vi "After Launch Init Core.vi"(8 "error in (no error)":errorcluster, 11 "CS++Scope in":refnum<class "CS++Scope.lvclass">) -> (0 "error out":errorcluster, 3 "CS++Scope out":refnum<class "CS++Scope.lvclass">)   [LabVIEW 2015, in "CS++Scope.lvlib" / "CS++Scope.lvclass"]
doc: "Use <b>Pre Launch init.vi</b> method for sanity checks that are supposed to prevent the actor from launching if they fail. Use <B>this</B> method instead to initialize this actor when it has been activated. A corresponding high priority message will become dispatched before the <B>Actor Core.vi</b> is called.\n\n<b>Derived classed should call the parent methode first</b> and their own initialization code after.\n\nRefer also to the ongoing discussion at https://decibel.ni.com/content/message/57394#57394."
uses:
  CS++Scope.lvclass
  CSPP_Core/Classes/CS++ProcessVariables/ProcessVariable/PV.lvclass
  <vilib>/ActorFramework/Actor/Actor.lvclass
  CSPP_Core/Classes/CS++ProcessVariables/PVConnection/PVConnection.lvclass
  CSPP_Core/Actors/CS++DeviceActor/CS++DeviceActor.lvclass
  <vilib>/ActorFramework/Batch Msg/Batch Msg.lvclass
  CS++Scope Messages/Configure Acquisition Type Msg/Configure Acquisition Type Msg.lvclass
  CS++Scope Messages/Configure Acquisition Record Msg/Configure Acquisition Record Msg.lvclass
  CS++Scope Messages/Configure Channel Msg/Configure Channel Msg.lvclass
  CS++Scope Messages/Configure Trigger Msg/Configure Trigger Msg.lvclass
  CS++Scope Messages/Configure Trigger Modifier [TM] Msg/Configure Trigger Modifier [TM] Msg.lvclass
  CS++Scope Messages/Configure Edge Trigger Source Msg/Configure Edge Trigger Source Msg.lvclass
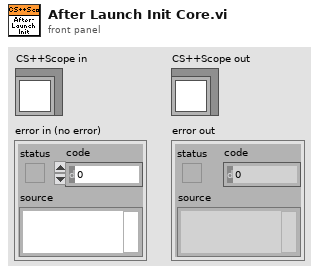
[diagram p1: front panel]
types:
  T1 = cluster{"Read Access":enum8{"Allowed", "Required", "None"}, "Write Access":enum8{"Allowed", "Required", "None"}}
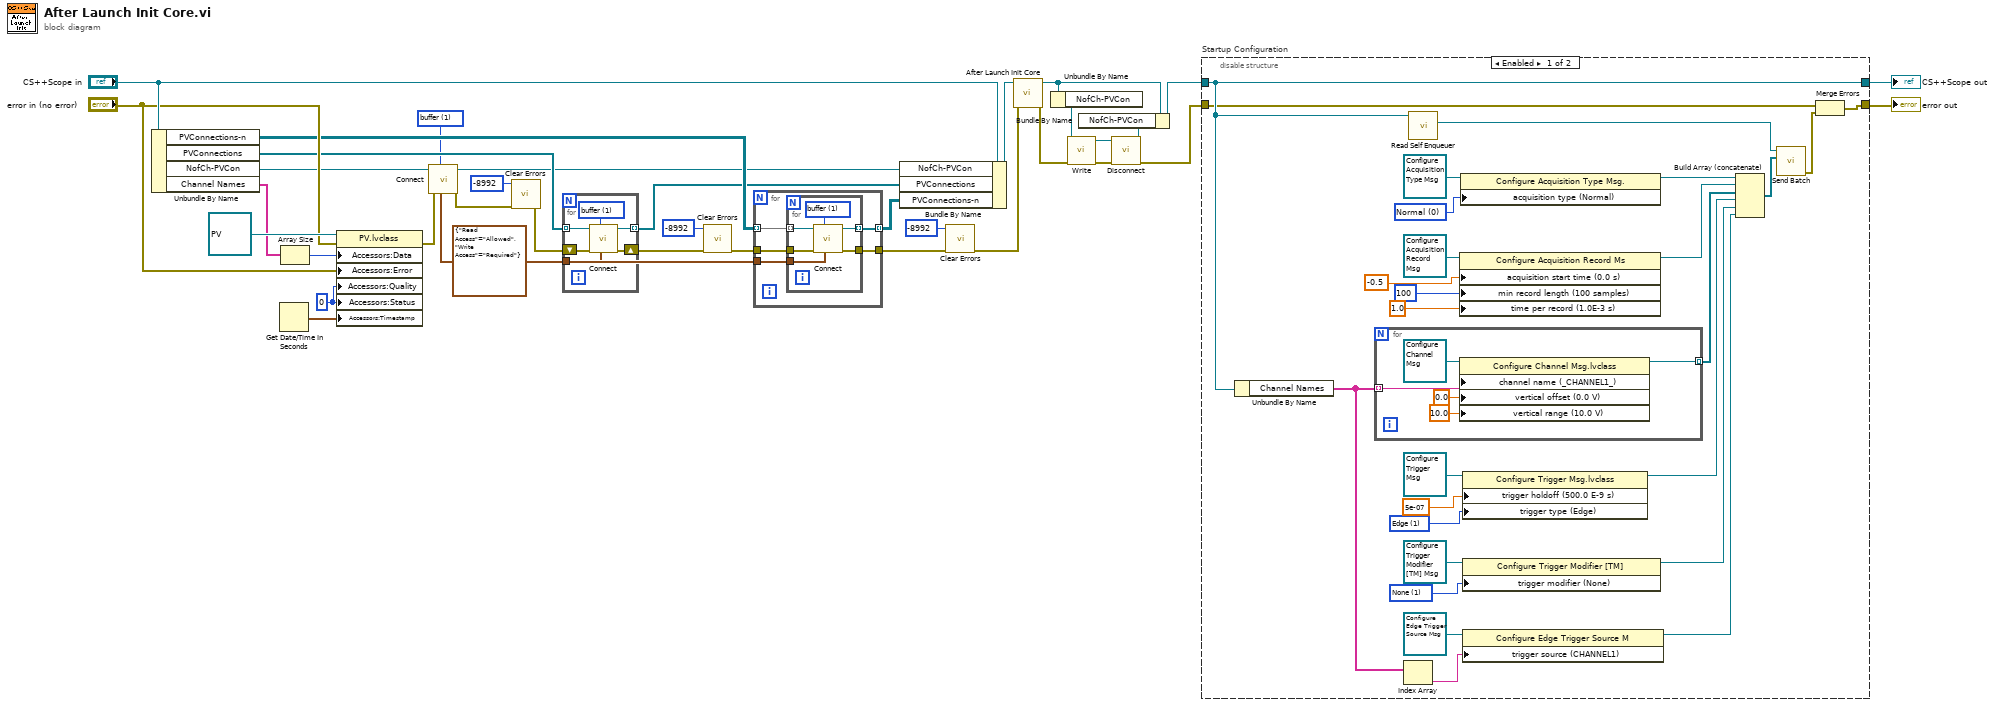
[diagram p0: block diagram]
diagram:
  w15 = u16 1 items=["commit", "buffer"] ("Mode (commit)")
  w20 = T1 {"Read Access"=enum."Allowed", "Write Access"=enum."Required"} ("Access (R/W allowed)")
  w26 = 0 ("Status")
  n1 = Unbundle By Name("CS++Scope in") -> ("PVConnections-n"=w29:refnum<class "PVConnection.lvclass">[][], "PVConnections"=w30:refnum<class "PVConnection.lvclass">[], "NofCh-PVCon"=w32:refnum<class "PVConnection.lvclass">, "Channel Names"=w23:string[])
  n2 = Get Date/Time In Seconds() -> (seconds since 1Jan1904=w25:timestamp)
  n3 = Array Size(array=w23) -> (size(s)=w24:i32)
  n4 = property class="PV.lvclass"(reference=refnum<class "PV.lvclass"> refnum ("CS++ProcessVariables.lvlib:PV.lvclass"), error in="error in (no error)", "Accessors:Data"=w24, "Accessors:Error"="error in (no error)", "Accessors:Quality"=w26, "Accessors:Status"=w26, "Accessors:Timestamp"=w25) -> (error out=w31:errorcluster)  [unwired: 1 out]
  n5 = call "Connect.vi"("Access (R/W allowed)"=w20, "Mode (buffer)"=w15, "Error In"=w31, "PVConnection in"=w32) -> ("Error Out"=w13:errorcluster, "PVConnection out"=w16:refnum<class "PVConnection.lvclass">)  [unwired: 6 in]
  n6 = call <vilib>:"Clear Errors.vi"("error in (no error)"=w13, "specific error code to clear (0: all)"=-8992) -> ("error out"=w12:errorcluster)  [unwired: 4 in, 1 out]
  n7 = for {
    tunnel: w30 -> [w42] mode=indexing
    shift-right: [w40] -> w10
    shift-left: w12 -> [w41]
    tunnel: [w39] -> w27 mode=indexing
    tunnel: w20 -> [w38]
    w37 = u16 1 items=["commit", "buffer"] ("Mode (commit)")
    n8 = call "Connect.vi"("Access (R/W allowed)"=w38, "Mode (buffer)"=w37, "Error In"=w41, "PVConnection in"=w42) -> ("Error Out"=w40:errorcluster, "PVConnection out"=w39:refnum<class "PVConnection.lvclass">)  [unwired: 6 in]
  }
  n9 = call <vilib>:"Clear Errors.vi"("error in (no error)"=w10, "specific error code to clear (0: all)"=-8992) -> ("error out"=w9:errorcluster)  [unwired: 4 in, 1 out]
  n10 = for {
    tunnel: w29 -> [w47] mode=indexing
    tunnel: [w44] -> w28 mode=indexing
    tunnel: w20 -> [w43]
    tunnel: w9 -> [w46]
    tunnel: [w45] -> w18
    n11 = for {
      tunnel: w47 -> [w53] mode=indexing
      tunnel: [w50] -> w44 mode=indexing
      tunnel: w43 -> [w49]
      tunnel: w46 -> [w52]
      tunnel: [w51] -> w45
      w48 = u16 1 items=["commit", "buffer"] ("Mode (commit)")
      n12 = call "Connect.vi"("Access (R/W allowed)"=w49, "Mode (buffer)"=w48, "Error In"=w52, "PVConnection in"=w53) -> ("Error Out"=w51:errorcluster, "PVConnection out"=w50:refnum<class "PVConnection.lvclass">)  [unwired: 6 in]
    }
  }
  n13 = Bundle By Name(cluster="CS++Scope in", "NofCh-PVCon"=w16, "PVConnections"=w27, "PVConnections-n"=w28) -> (w35:refnum<class "CS++Scope.lvclass">)
  n14 = call <vilib>:"Clear Errors.vi"("error in (no error)"=w18, "specific error code to clear (0: all)"=-8992) -> ("error out"=w17:errorcluster)  [unwired: 4 in, 1 out]
  n15 = call-parent "After Launch Init Core.vi"("error in (no error)"=w17, "CS++DeviceActor in"=w35) -> ("error out"=w5:errorcluster, "CS++DeviceActor out"=w3:refnum<class "CS++Scope.lvclass">)  [unwired: 8 in]
  n16 = Unbundle By Name(w3) -> ("NofCh-PVCon"=w6:refnum<class "PVConnection.lvclass">)
  n17 = call "Write.vi"("error in (no error)"=w5, "PVConnection in"=w6) -> ("error out"=w7:errorcluster, "PVConnection out"=w8:refnum<class "PVConnection.lvclass">)  [unwired: 8 in]
  n18 = call "Disconnect.vi"("error in (no error)"=w7, "PVConnection in"=w8) -> ("error out"=w4:errorcluster, "PVConnection out"=w1:refnum<class "PVConnection.lvclass">)  [unwired: 8 in]
  n19 = Bundle By Name(cluster=w3, "NofCh-PVCon"=w1) -> (w2:refnum<class "CS++Scope.lvclass">)
  n20 = disable-structure "Startup Configuration" shown="Enabled" {
    disable-tunnel: w4 -> [w54 w85]
    disable-tunnel: [w56 w85] -> w21
    disable-tunnel: [w57 w86] -> w22
    disable-tunnel: w2 -> [w57 w86]
    frame Enabled {
      w68 = 1 items=["None"=1, "Auto"=2, "Auto Level"=3] ("trigger modifier (None)")
      w66 = 1 items=["Edge"=1, "TV"=5, "Runt"=3, "Glitch"=4, "Width"=2, "AC Line"=7, "Immediate"=6] ("trigger type (Edge)")
      w59 = 0 items=["Normal", "Peak Detect", "High Resolution", "Envelope", "Average"] ("acquisition type (Normal)")
      n21 = Unbundle By Name(w57) -> ("Channel Names"=w79:string[])
      n22 = for {
        tunnel: [w83] -> w73 mode=indexing
        tunnel: w79 -> [w82] mode=indexing
        n23 = property class="Configure Channel Msg.lvclass"(reference=refnum<class "Configure Channel Msg.lvclass"> refnum ("CS++Scope.lvlib:Configure Channel Msg.lvclass"), "channel name (_CHANNEL1_)"=w82, "vertical offset (0.0 V)"=dbl[unit] 0.0, "vertical range (10.0 V)"=dbl[unit] 10.0) -> (reference out=w83:refnum<class "Configure Channel Msg.lvclass">)  [unwired: 1 in, 1 out]
      }
      n24 = Index Array(array=w79) -> (element=w70:string)  [unwired: 1 in]
      n25 = call <vilib>:"Read Self Enqueuer.vi"("Actor"=w57) -> ("Self Enqueuer"=w78:refnum<class "Message Enqueuer.lvclass">)  [unwired: 10 in]
      n26 = property class="Configure Acquisition Record Ms"(reference=refnum<class "Configure Acquisition Record Msg.lvclass"> refnum ("CS++Scope.lvlib:Configure Acquisition Record Msg.lvclass"), "acquisition start time (0.0 s)"=dbl[unit] -0.5, "min record length (100 samples)"=100, "time per record (1.0E-3 s)"=dbl[unit] 1.0) -> (reference out=w72:refnum<class "Configure Acquisition Record Msg.lvclass">)  [unwired: 1 in, 1 out]
      n27 = property class="Configure Acquisition Type Msg."(reference=refnum<class "Configure Acquisition Type Msg.lvclass"> refnum ("CS++Scope.lvlib:Configure Acquisition Type Msg.lvclass"), "acquisition type (Normal)"=w59) -> (reference out=w71:refnum<class "Configure Acquisition Type Msg.lvclass">)  [unwired: 1 in, 1 out]
      n28 = property class="Configure Trigger Msg.lvclass"(reference=refnum<class "Configure Trigger Msg.lvclass"> refnum ("CS++Scope.lvlib:Configure Trigger Msg.lvclass"), "trigger holdoff (500.0 E-9 s)"=dbl[unit] 5e-07, "trigger type (Edge)"=w66) -> (reference out=w74:refnum<class "Configure Trigger Msg.lvclass">)  [unwired: 1 in, 1 out]
      n29 = property class="Configure Trigger Modifier [TM]"(reference=refnum<class "Configure Trigger Modifier [TM] Msg.lvclass"> refnum ("CS++Scope.lvlib:Configure Trigger Modifier [TM] Msg.lvclass"), "trigger modifier (None)"=w68) -> (reference out=w75:refnum<class "Configure Trigger Modifier [TM] Msg.lvclass">)  [unwired: 1 in, 1 out]
      n30 = property class="Configure Edge Trigger Source M"(reference=refnum<class "Configure Edge Trigger Source Msg.lvclass"> refnum ("CS++Scope.lvlib:Configure Edge Trigger Source Msg.lvclass"), "trigger source (CHANNEL1)"=w70) -> (reference out=w76:refnum<class "Configure Edge Trigger Source Msg.lvclass">)  [unwired: 1 in, 1 out]
      n31 = Build Array (concatenate)(w71, w72, w73, w74, w75, w76) -> (w77:refnum<class "Message.lvclass">[])
      n32 = call <vilib>:"Send Batch.vi"("Messages Array"=w77, "Message Enqueuer"=w78) -> ("error out"=w55:errorcluster)  [unwired: 9 in]
      n33 = Merge Errors(w54, w55) -> (w56:errorcluster)
    }
    frame Disabled {
    }
  }
  "error out" <- w21
  "CS++Scope out" <- w22
